vi "MaxValuevi.vi"(1 "Numeric":dbl) -> (0 "Numeric 2":dbl)   [LabVIEW 2018]
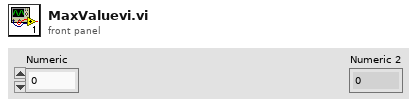
[diagram p1: front panel]
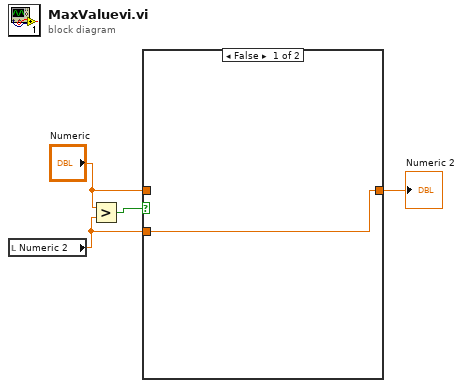
[diagram p0: block diagram]
diagram:
  n1 = local read "Numeric 2"() -> (w1:dbl)
  n2 = Greater?(x="Numeric", y=w1) -> (0:w4:bool)
  n3 = case shown="False" w4 {
    tunnel: "Numeric" -> [_ w6]
    tunnel: [w5 w6] -> w2
    tunnel: w1 -> [w5 _]
    frame False {
    }
    frame True {
    }
  }
  "Numeric 2" <- w2
